vi "624WPI_DashboardGetInfo.vi"(7 "Vision":u16(ring) items=["Camera Off", "USB Camera SW", "USB Camera HW", "IP Camera"], 8 "Binding Refnum":refnum<notifier>, 9 "Window Mode Notifier":refnum<notifier>, 11 "TCP Cnx":refnum<k5>) -> (0 "Power and Errors":T2, 1 "Robot Metrics":T3, 2 "Status Info":T5, 3 "Control Info":T4 {"Team Station" items=["Red 1", "Red 2", "Red 3", "Blue 1", "Blue 2", "Blue 3"]}, 4 "Robot Mode":T1(ring), 5 "Process?":bool, 6 "Custom Dashboard Data":string)   [LabVIEW 2014]
uses:
  Dashboard Hijack Data.ctl
  <vilib>/Rock Robotics/WPI/Dashboard/WPI_DashboardLogging Global.vi
panel:
  # "CAN Metrics\nJS HID Outputs\nFree Mem"
  # "Need to merge in TCP info too"
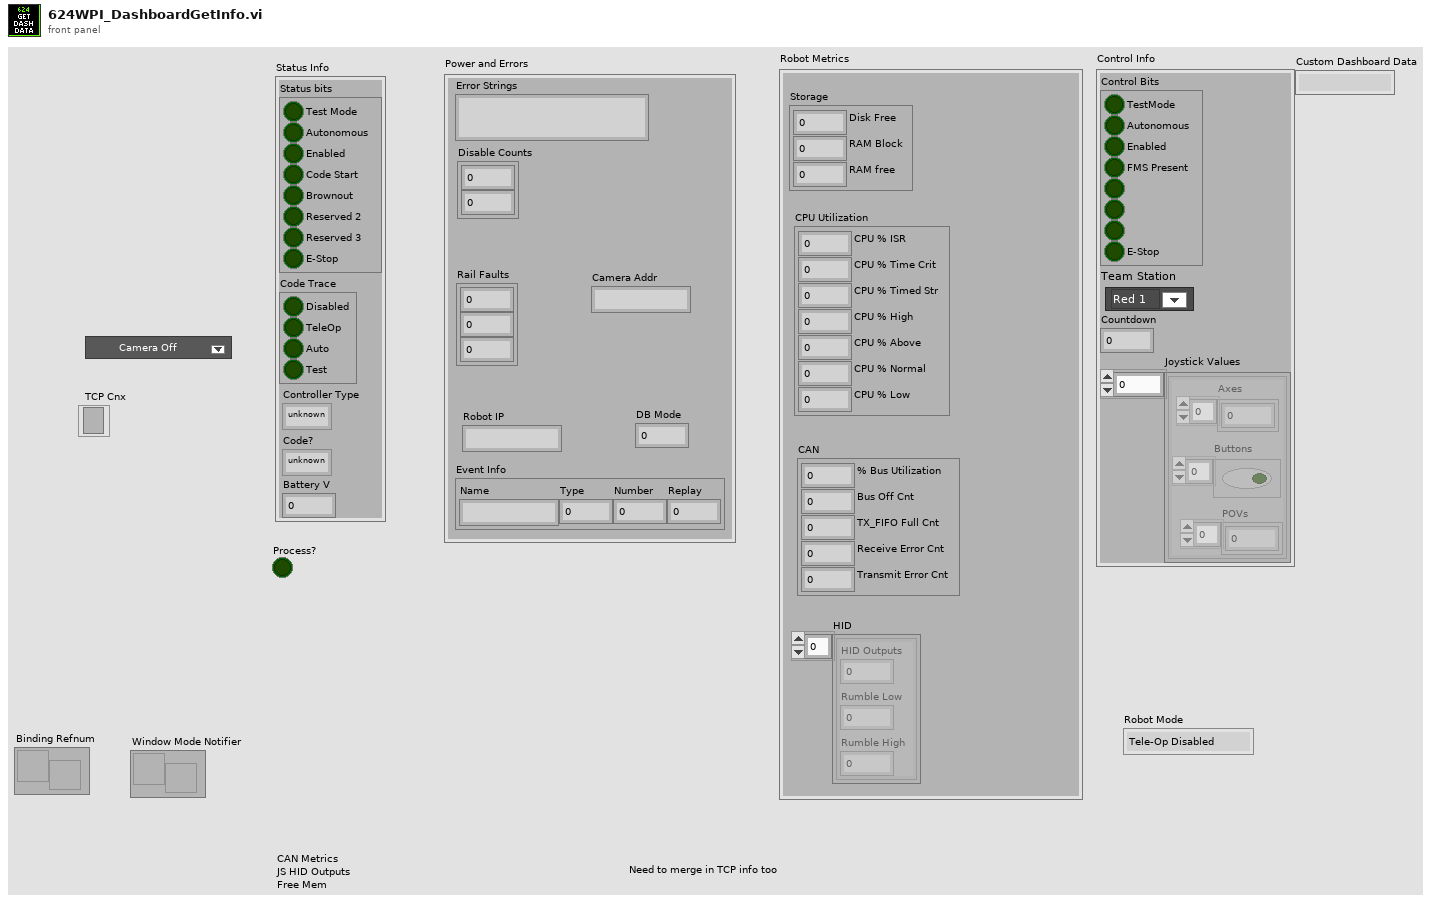
[diagram p1: front panel]
types:
  T1 = enum8{"Tele-Op Disabled", "Tele-Op Enabled", "Auto Disabled", "Auto Enabled", "Test Disabled", "Test Enabled", "Disconnected", "No Code", "E-Stop"}
  T2 = cluster{"Error Strings":string, "Disable Counts":cluster{u16, u16}, "Rail Faults":cluster{u16, u16, u16}, "Robot IP":string, "DB Mode":u8, "Event Info":cluster{"Name":string, "Type":u8, "Number":u16, "Replay":u8}, "Camera Addr":string}
  T3 = cluster{"Storage":cluster{"Disk Free":u64, "RAM Block":u32, "RAM free":u32}, "CPU Utilization":cluster{"CPU % ISR":sgl, "CPU % Time Crit":sgl, "CPU % Timed Str":sgl, "CPU % High":sgl, "CPU % Above":sgl, "CPU % Normal":sgl, "CPU % Low":sgl}, "CAN":cluster{"% Bus Utilization":sgl, "Bus Off Cnt":u32, "TX_FIFO Full Cnt":u32, "Receive Error Cnt":u8, "Transmit Error Cnt":u8}, "HID":cluster{"HID Outputs":u32, "Rumble Low":u16, "Rumble High":u16}[]}
  T4 = cluster{"Control Bits":cluster{"TestMode":bool, "Autonomous":bool, "Enabled":bool, "FMS Present":bool, bool, bool, bool, "E-Stop":bool}, "Team Station ":u8, "Countdown":sgl, "Joystick Values":cluster{"Axes":dbl[], "Buttons":bool[], "POVs":i16[]}[]}
  T5 = cluster{"Status bits":cluster{"Test Mode":bool, "Autonomous":bool, "Enabled":bool, "Code Start":bool, "Brownout":bool, "Reserved 2":bool, "Reserved 3":bool, "E-Stop":bool}, "Code Trace":cluster{"Disabled":bool, "TeleOp":bool, "Auto":bool, "Test":bool}, "Controller Type":enum16{"unknown", "cRIO", "roboRio"}, "Code?":enum16{"unknown", "noCode", "code"}, "Battery V":dbl}
  T6 = typedef "Dashboard Hijack Data.ctl" = cluster{"UDP Status string":string, "Extra data string":string}
  T7 = cluster{"TestMode":bool, "Autonomous":bool, "Enabled":bool, "FMS Present":bool, bool, bool, bool, "E-Stop":bool}
  T8 = enum16{"Standard", "Buffered", "CRLF", "Immediate"}
  T9 = cluster{"UDP Status":string, "TCP":string, "UDP Control":string}
  T10 = cluster{cluster{"Disk Free":u64, "RAM Block":u32, "RAM free":u32}, cluster{"CPU Load ISR":sgl, "CPU Load Time Critical Pr":sgl, "CPU Load Timed Str Pr":sgl, "CPU Load High Pr":sgl, "CPU Load Above Normal Pr":sgl, "CPU Load Normal Pr":sgl, "CPU Load Low Pr":sgl}, cluster{"% Bus Utilization":sgl, "Bus Off Cnt":u32, "TX_FIFO Full Cnt":u32, "Receive Error Cnt":u8, "Transmit Error Cnt":u8}, cluster{"HID Outputs":u32, "Rumble Low":u16, "Rumble High":u16}[]}
  T11 = cluster{"Status":cluster{"Test Mode":bool, "Autonomous":bool, "Enabled":bool, "Code Start":bool, "Brownout":bool, "Reserved 2":bool, "Reserved 3":bool, "E-Stop":bool}, cluster{bool, bool, bool, bool}, "ctrl":enum16{"unknown", "cRIO", "roboRio"}, "code?":enum16{"unknown", "noCode", "code"}, dbl}
  T12 = cluster{"Boolean array":cluster{"Boolean array[0]":bool, "Boolean array[1]":bool, "Boolean array[2]":bool, "Boolean array[3]":bool, "Boolean array[4]":bool, "Boolean array[5]":bool, "Boolean array[6]":bool, "Boolean array[7]":bool}, u8, "Countdown":sgl, cluster{dbl[], bool[], i16[]}[]}
  T13 = cluster{"Error Strings":string, "Disable Counts":cluster{u16, u16}, "Rail Faults":cluster{u16, u16, u16}, "Robot IP":string, "Mode":u8, "Event Info":cluster{"Name":string, "Type":u8, "Number":u16, "Replay":u8}, "Robot IP":string}
  T14 = cluster{"Boolean array[0]":bool, "Boolean array[1]":bool, "Boolean array[2]":bool, "Boolean array[3]":bool, "Boolean array[4]":bool, "Boolean array[5]":bool, "Boolean array[6]":bool, "Boolean array[7]":bool}
  T15 = typedef "Protocol Operations.ctl" = enum16{"Unknown", "Keep Alive", "Hello", "Version not supported", "Hello Complete", "Assign", "Update", "No Op"}
  T16 = typedef "Field Data.ctl" = cluster{"Dbl":dbl, "String":string, "Type":T17, "Boolean":bool, "Sequence #":T18}
  T17 = typedef "Field Type.ctl" = enum8{"Invalid", "Bool", "Numeric", "String", "Boolean Array", "Numeric Array", "String Array"}
  T18 = typedef "Sequence.ctl" = u16
  T19 = cluster{"Operation":T15, "Name":string, "Field Value":T16}[]
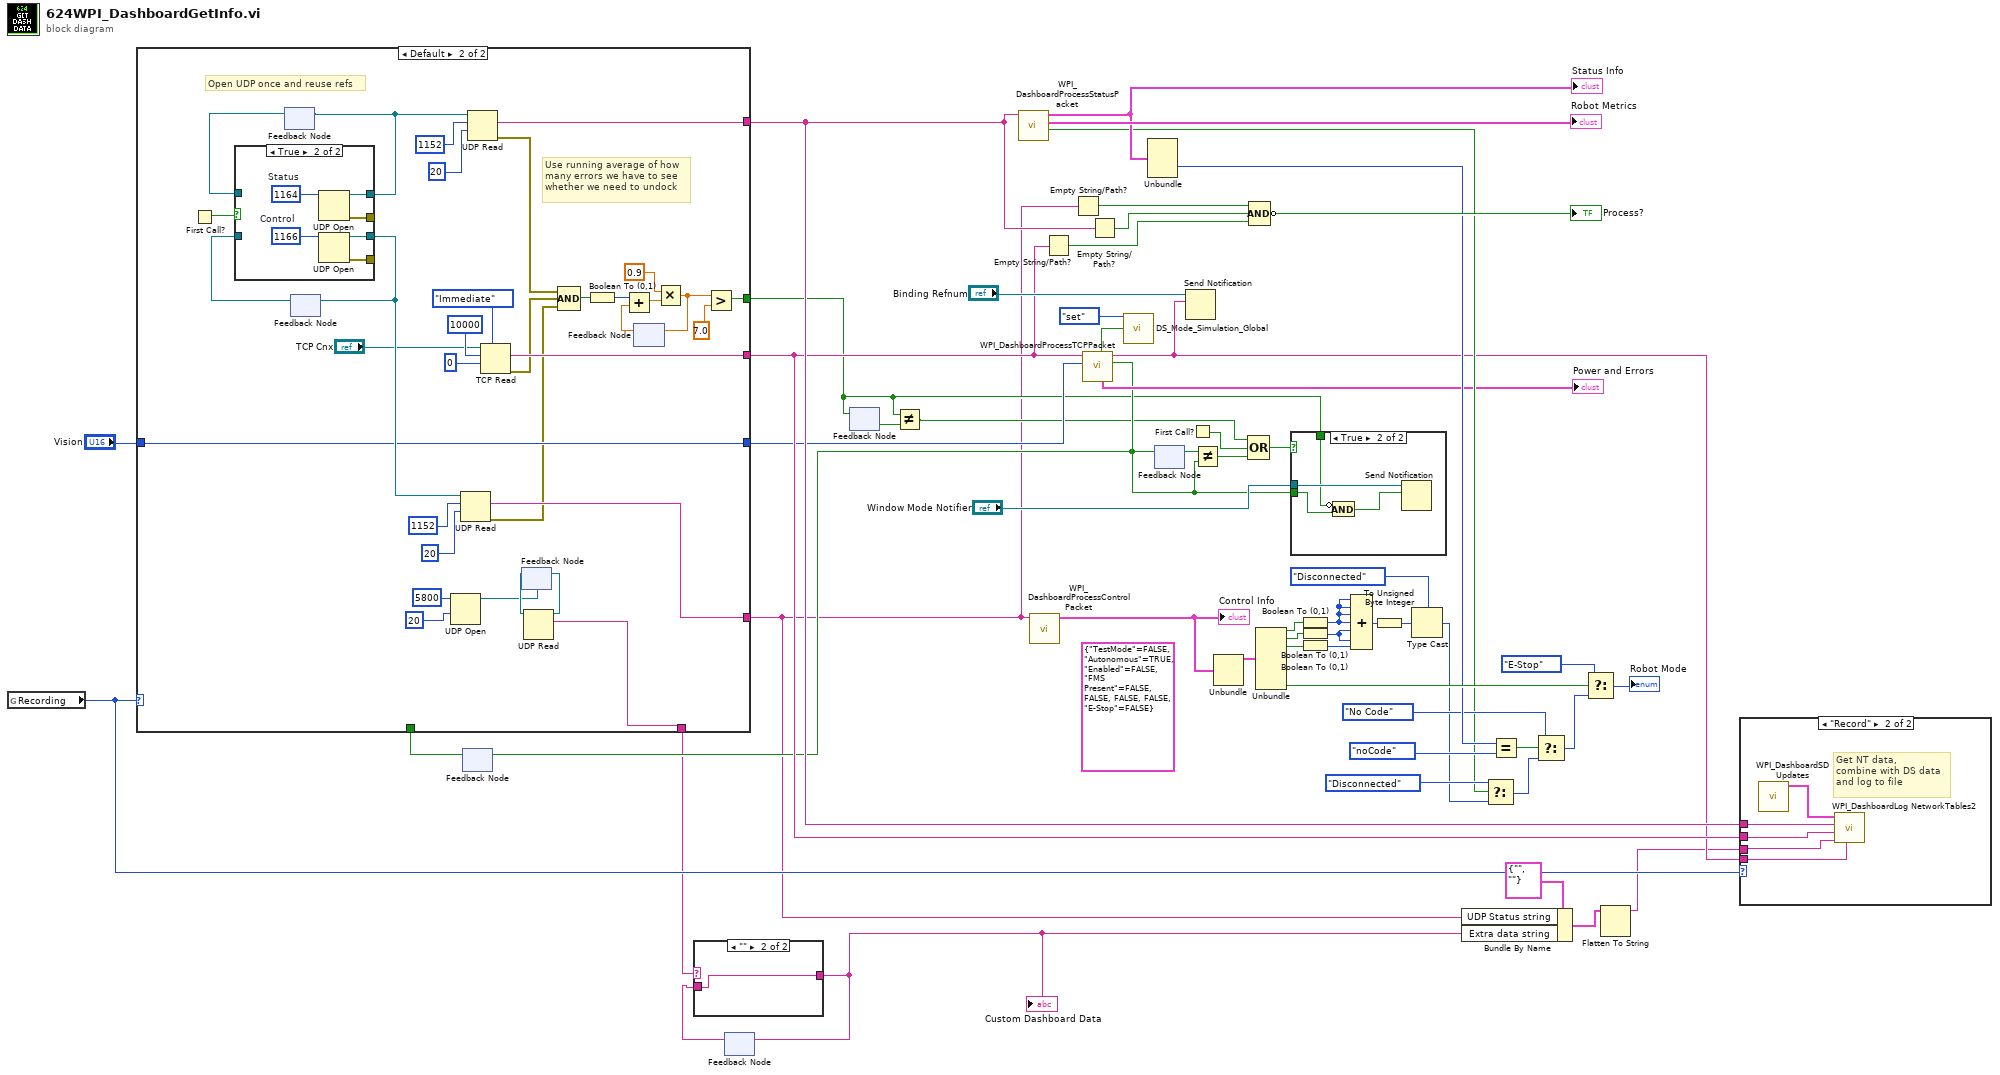
[diagram p0: block diagram]
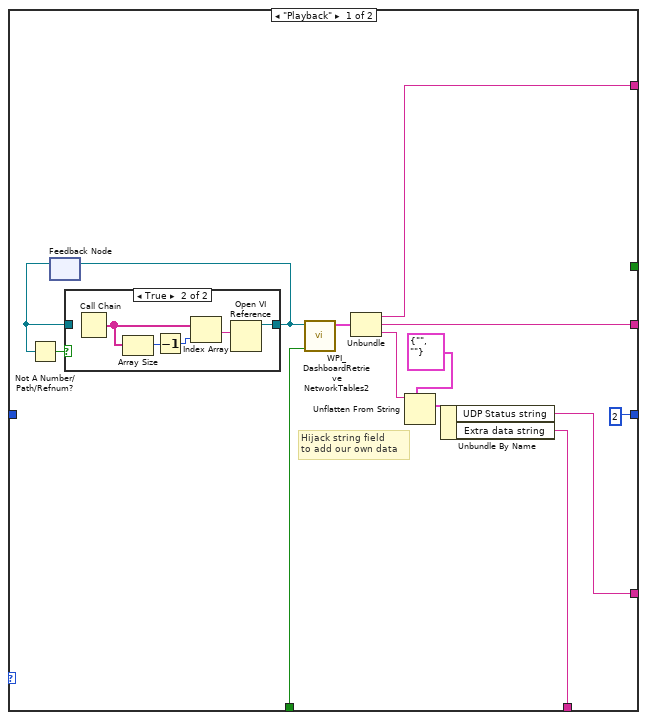
[diagram p4: hidden frame]
diagram:
  (unwired) T7 {"TestMode"=FALSE, "Autonomous"=TRUE, "Enabled"=FALSE, "FMS Present"=FALSE, FALSE, FALSE, FALSE, "E-Stop"=FALSE} ("Control Bits")
  n1 = global read "WPI_DashboardLogging Global.vi" "Recording"() -> (w11:enum32{"Stop", "Record", "Playback"})
  n2 = feedback #1() -> (w14:bool)  [unwired: 1 in]
  n3 = case shown="Default" w11 {
    tunnel: [w58 w102] -> w6
    tunnel: [w65 w101] -> w19
    tunnel: [w64 w100] -> w18
    tunnel: w14 -> [w63 _]
    tunnel: "Vision" -> [_ w93]
    tunnel: [2 ("timeout ms (25000)") w93] -> w12
    tunnel: [_ w82] -> w10
    tunnel: [w57 w76] -> w3
    frame "Playback" {
      # "Hijack string field\nto add our own data"
      n4 = feedback #2() -> (w69:refnum<vi>)  [unwired: 1 in]
      n5 = Not A Number/Path/Refnum?(number/path/refnum=w69) -> (NaN/Path/Refnum?=w68:bool)
      n6 = case shown="True" w68 {
        tunnel: w69 -> [w70 _]
        tunnel: [w70 w74] -> w66
        frame False {
        }
        frame True {
          n7 = Call Chain() -> (call chain=w73:string[])
          n8 = Array Size(array=w73) -> (size(s)=w72:i32)
          n9 = Decrement(x=w72) -> (x-1=w71:i32)
          n10 = Index Array(array=w73, index=w71) -> (element=w75:string)
          n11 = Open VI Reference(vi path=w75) -> (vi reference=w74:refnum<vi>)  [unwired: 5 in, 1 out]
        }
      }
      n12 = feedback-in #2(w66) -> ()
      n13 = call <vilib>:"WPI_DashboardRetrieve NetworkTables2.vi"("Docked Window"=w63, "VI Refnum"=w66) -> ("Strings"=w67:T9)  [unwired: 9 in]
      n14 = Unbundle(w67) -> ("UDP Status"=w65:string, "TCP"=w64:string, "UDP Control"=w61:string)
      n15 = Unflatten From String(type=T6 {"UDP Status string"="", "Extra data string"=""} ("Dashboard Data Hijack"), binary string=w61) -> (value=w59:T6)  [unwired: 3 in, 2 out]
      n16 = Unbundle By Name(w59) -> ("UDP Status string"=w58:string, "Extra data string"=w57:string)
    }
    frame Default {
      # "Use running average of how\nmany errors we have to see\nwhether we need to undock"
      # "Open UDP once and reuse refs"
      n17 = First Call?() -> (First Call?: T/F=w99:bool)
      n18 = feedback #3() -> (w97:refnum<k16>)  [unwired: 1 in]
      n19 = feedback #4() -> (w95:refnum<k16>)  [unwired: 1 in]
      n20 = case shown="True" w99 {
        tunnel: [w111 w115] -> w98
        tunnel: [_ w114] -> _
        tunnel: [w110 w113] -> w96
        tunnel: [_ w112] -> _
        tunnel: w97 -> [w111 _]
        tunnel: w95 -> [w110 _]
        frame False {
        }
        frame True {
          w116 = u16 1166  # Control
          w117 = u16 1164  # Status
          n21 = UDP Open(11:w117) -> (port=w115:refnum<k16>, 0:w114:errorcluster)  [unwired: 2 in, 3 out]
          n22 = UDP Open(11:w116) -> (port=w113:refnum<k16>, 0:w112:errorcluster)  [unwired: 2 in, 3 out]
        }
      }
      n23 = feedback-in #3(w98) -> ()
      n24 = feedback-in #4(w96) -> ()
      n25 = UDP Open(9:20 ("timeout ms (25000)"), 11:u16 5800 ("port")) -> (port=w78:refnum<k16>)  [unwired: 3 in, 2 out]
      n26 = UDP Read(connection ID=w96, max size (548)=1152, timeout ms (25000)=20 ("length (rest)")) -> (data out=w102:string, error out=w90:errorcluster)  [unwired: 1 in, 3 out]
      n27 = UDP Read(connection ID=w98, max size (548)=1152, timeout ms (25000)=20 ("length (rest)")) -> (data out=w101:string, error out=w92:errorcluster)  [unwired: 1 in, 3 out]
      n28 = TCP Read(connection ID="TCP Cnx", bytes to read=10000 ("timeout ms (25000)"), 7:T8."Immediate" ("mode (standard)"), 9:0 ("timeout ms (25000)")) -> (data out=w100:string, error out=w91:errorcluster)  [unwired: 1 in, 1 out]
      n29 = feedback #5(w78) -> (w79:refnum<k16>)
      n30 = UDP Read(connection ID=w79) -> (data out=w76:string, 3:w80:refnum<k16>)  [unwired: 3 in, 3 out]
      n31 = feedback-in #5(w80) -> ()
      n32 = Compound Arithmetic op=AND(w92, w91, w90) -> (w89:bool)
      n33 = Boolean To (0,1)(Boolean=w89) -> (0, 1=w88:i16)
      n34 = feedback #6() -> (w87:dbl)  [unwired: 1 in]
      n35 = Add(x=w88, y=w87) -> (x+y=w86:dbl)
      n36 = Multiply(x=0.9 ("timeout ms (25000)"), y=w86) -> (x*y=w84:dbl)
      n37 = feedback-in #6(w84) -> ()
      n38 = Greater?(x=w84, y=7.0 ("timeout ms (25000)")) -> (0:w82:bool)
    }
  }
  n39 = feedback #7() -> (w2:string)  [unwired: 1 in]
  n40 = case shown="\"\"" w3 {
    selector: w3 -> [w118 _]
    tunnel: [w118 w119] -> w1
    tunnel: w2 -> [_ w119]
    frame Default {
    }
    frame "" {
    }
  }
  "Custom Dashboard Data" <- w1
  n41 = feedback-in #7(w1) -> ()
  n42 = feedback #8() -> (w9:bool)  [unwired: 1 in]
  n43 = feedback-in #8(w10) -> ()
  n44 = Not Equal?(x=w10, y=w9) -> (x != y?=w8:bool)
  n45 = call <vilib>:"WPI_DashboardProcessStatusPacket.vi"("data in"=w19) -> ("Disconnected"=w22:bool, "Robot Metrics"=→"Robot Metrics":T10, "Status Cluster"=w36:T11)  [unwired: 8 in]
  "Status Info" <- w36
  n46 = call <vilib>:"WPI_DashboardProcessControlPacket.vi"("data in"=w6) -> ("Control Info"=w44:T12)  [unwired: 10 in]
  "Control Info" <- w44
  n47 = Empty String/Path?(string/path=w18) -> (empty?=w54:bool)
  n48 = Empty String/Path?(string/path=w6) -> (empty?=w52:bool)
  n49 = call <vilib>:"WPI_DashboardProcessTCPPacket.vi"("Vision"=w12, "data in"=w18) -> ("Docked"=w15:bool, "Robot IP"=w16:string, "Power and Errors"=→"Power and Errors":T13, "Simulated"=w20:bool)  [unwired: 5 in, 1 out]
  n50 = feedback-in #1(w15) -> ()
  n51 = Empty String/Path?(string/path=w19) -> (empty?=w53:bool)
  n52 = call <vilib>:"DS_Mode_Simulation_Global.vi"("menu"=enum16{"set", "get"}."set", "simulated? in"=w20) -> ()  [unwired: 12 in, 2 out]
  n53 = Unbundle(w36) -> ("code?"=w32:enum16{"unknown", "noCode", "code"})  [unwired: 4 out]
  n54 = feedback #9() -> (w47:bool)  [unwired: 1 in]
  n55 = feedback-in #9(w15) -> ()
  n56 = Send Notification(notification=w16, notifier="Binding Refnum") -> ()  [unwired: 1 in, 2 out]
  n57 = First Call?() -> (First Call?: T/F=w49:bool)
  n58 = Not Equal?(x=w47, y=w15) -> (x != y?=w48:bool)
  n59 = Unbundle(w44) -> ("Boolean array"=w43:T14)  [unwired: 3 out]
  n60 = Compound Arithmetic op=OR(w8, w49, w48) -> (w50:bool)
  n61 = Compound Arithmetic op=AND(w52, w53, w54) -> (invert →"Process?":bool)
  n62 = Unbundle(w43) -> ("Boolean array[0]"=w38:bool, "Boolean array[1]"=w39:bool, "Boolean array[2]"=w41:bool, "Boolean array[7]"=w35:bool)  [unwired: 4 out]
  n63 = case shown="True" w50 {
    tunnel: "Window Mode Notifier" -> [_ w123]
    tunnel: w15 -> [_ w121]
    tunnel: w10 -> [_ w122]
    frame False {
    }
    frame True {
      n64 = Compound Arithmetic op=AND(invert w122, w121) -> (w120:bool)
      n65 = Send Notification(notification=w120, notifier=w123) -> ()  [unwired: 1 in, 2 out]
    }
  }
  n66 = Boolean To (0,1)(Boolean=w38) -> (0, 1=w37:i16)
  n67 = Boolean To (0,1)(Boolean=w39) -> (0, 1=w40:i16)
  n68 = Boolean To (0,1)(Boolean=w41) -> (0, 1=w42:i16)
  n69 = Compound Arithmetic op=ADD(w37, w37, w37, w37, w40, w40, w42) -> (w26:i16)
  n70 = To Unsigned Byte Integer(number=w26) -> (unsigned 8bit integer=w21:u8)
  n71 = Type Cast(type=T1."Disconnected" ("Mode"), x=w21) -> (*(type *) &x=w25:T1)
  n72 = Bundle By Name(cluster=T6 {"UDP Status string"="", "Extra data string"=""} ("Dashboard Data Hijack"), "UDP Status string"=w6, "Extra data string"=w1) -> (w5:T6)
  n73 = Select(t=T1."Disconnected" ("Mode"), s=w22, f=w25) -> (s? t:f=w28:T1)
  n74 = Equal?(x=w32, y=enum16{"unknown", "noCode", "code"}."noCode" ("code?")) -> (x = y?=w31:bool)
  n75 = Select(t=T1."No Code" ("Mode"), s=w31, f=w28) -> (s? t:f=w30:T1)
  n76 = Select(t=T1."E-Stop" ("Mode"), s=w35, f=w30) -> (s? t:f=→"Robot Mode":T1)
  n77 = Flatten To String(anything=w5) -> (data string=w4:string)  [unwired: 3 in, 2 out]
  n78 = case shown="\"Record\"" w11 {
    tunnel: w19 -> [_ w125]
    tunnel: w18 -> [_ w126]
    tunnel: w4 -> [_ w127]
    tunnel: w16 -> [_ w124]
    frame Default {
    }
    frame "Record" {
      # "Get NT data,\ncombine with DS data\nand log to file"
      n79 = call <vilib>:"WPI_DashboardSD Updates.vi"() -> ("Collected Data"=w128:T19)  [unwired: 11 in]
      n80 = call <vilib>:"WPI_DashboardLog NetworkTables2.vi"("Robot IP"=w124, "UDP Control"=w127, "TCP"=w126, "UDP Status"=w125, "NT Data Values"=w128) -> ()  [unwired: 7 in]
    }
  }
